vi "Log_Processed.vi"(10 "Array in":sgl[](array[numeric]), 11 "Byte Stream File in":refnum<file>) -> (3 "Byte Stream File out":refnum<file>)   [LabVIEW 2020]
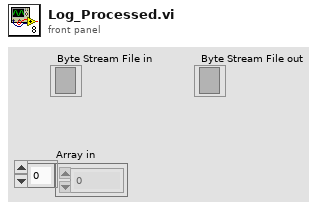
[diagram p1: front panel]
types:
  T1 = cluster{"Array in[0]":sgl, "Array in[1]":sgl, "Array in[2]":sgl, "Array in[3]":sgl, "Array in[4]":sgl, "Array in[5]":sgl, "Array in[6]":sgl, "Array in[7]":sgl, "Array in[8]":sgl}
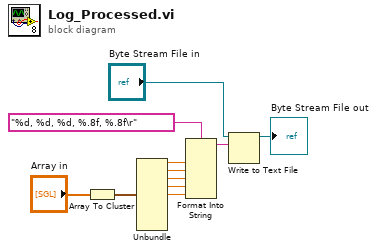
[diagram p0: block diagram]
diagram:
  n1 = Array To Cluster(array="Array in") -> (cluster=w2:T1)
  n2 = Unbundle(w2) -> ("Array in[0]"=w3:sgl, "Array in[1]"=w4:sgl, "Array in[2]"=w5:sgl, "Array in[3]"=w6:sgl, "Array in[4]"=w7:sgl)  [unwired: 4 out]
  n3 = Format Into String(format string="%d, %d, %d, %.8f, %.8f\r", w3, w4, w5, w6, w7) -> (resulting string=w9:string)  [unwired: 2 in, 1 out]
  n4 = Write to Text File(file (use dialog)="Byte Stream File in", text=w9) -> (refnum out=→"Byte Stream File out":refnum<file>)  [unwired: 2 in, 2 out]
